vi "Read Transfer Buffer.vi"(8 "error in":errorcluster, 10 "Transfer":refnum<class "Transfer.lvclass">, 11 "RDMA Transceiver in":refnum<class "RDMA Transceiver.lvclass">) -> (0 "error out":errorcluster, 1 "data":u8[](array[numeric]), 3 "RDMA Transceiver out":refnum<class "RDMA Transceiver.lvclass">)   [LabVIEW 2020, in "RDMA.lvlib" / "RDMA Transceiver.lvclass"]
uses:
  RDMA Transceiver.lvclass
  DSF Core.lvlibp/Classes/Transfer/Transfer.lvclass
  RDMA Transceiver.lvclass/RDMA Transceiver.ctl
  DSF Core.lvlibp/Classes/Buffer/Read Buffer 1D U8.vi
  DSF Core.lvlibp/Classes/Buffer/Buffer.lvclass
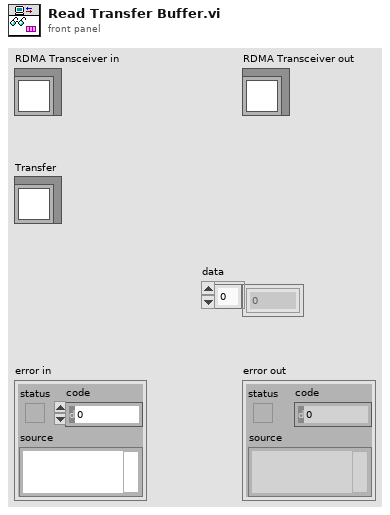
[diagram p1: front panel]
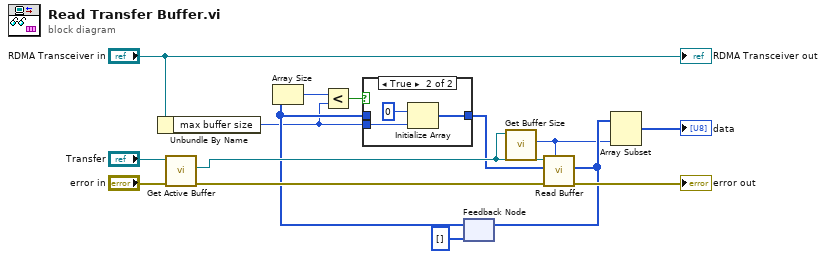
[diagram p0: block diagram]
diagram:
  n1 = Unbundle By Name("RDMA Transceiver in") -> ("max buffer size"=w3:i32)
  n2 = call "Get Active Buffer.vi"("error in (no error)"="error in", "Transfer in"="Transfer") -> ("error out"=w12:errorcluster, "Buffer"=w9:refnum<class "Buffer.lvclass">)  [unwired: 7 in, 1 out]
  n3 = feedback #1(u8[] []) -> (w5:u8[])
  n4 = Array Size(array=w5) -> (size(s)=w4:i32)
  n5 = Less?(x=w4, y=w3) -> (x < y?=w2:bool)
  n6 = case shown="True" w2 {
    tunnel: w5 -> [w16 _]
    tunnel: [w16 w19] -> w8
    tunnel: w3 -> [_ w17]
    frame False {
    }
    frame True {
      n7 = Initialize Array(u8 0 ("Numeric"), w17) -> (w19:u8[])
    }
  }
  n8 = call "Get Buffer Size.vi"("Buffer in"=w9) -> ("buffer size"=w6:u64)  [unwired: 9 in, 1 out]
  n9 = call-poly "Read Buffer.vi"("count (-1: rest)"=w6, "error in (no error)"=w12, "dst array in"=w8, "Buffer in"=w9) -> ("error out"=→"error out":errorcluster, "dst array out"=w7:u8[])  [unwired: 4 in, 2 out]
  n10 = feedback-in #1(w7) -> ()
  n11 = Array Subset(array=w7, length=w6) -> (→"data":u8[])  [unwired: 1 in]
  "RDMA Transceiver out" <- "RDMA Transceiver in"
